vi "EditOptions.vi"(8 "error in":errorcluster, 11 "node in":refnum<class "CEF_serializable node folder.lvclass">=refnum) -> (0 "error out":errorcluster, 1 "edit options":T1, 2 "subnodes class":T2, 3 "node out":refnum<class "CEF_serializable node folder.lvclass">)   [LabVIEW 2025, in "CEF_serializable node folder.lvclass"]
doc: "Contains the options for the Menu that will be displayed when doing right click on an item.\nThe sub nodes class configures which nodes can be added to this nodes\nAnd the edit options determine which options are available for the node.\nThis configuration is stored in this VI in case some dynamic configuration is required for the menu options or sub nodes.\nCopyright 2017 National Instruments Corporation\n\nLicensed under the Apache License, Version 2.0 (the \"License\"); you may not use this file except in compliance with the License. You may obtain a copy of the License at http://www.apache.org/licenses/LICENSE-2.0\nUnless required by applicable law or agreed to in writing, software distributed under the License is distributed on an \"AS IS\" BASIS, WITHOUT WARRANTIES OR CONDITIONS OF ANY KIND, either express or implied. See the License for the specific language governing permissions and limitations under the License."
uses:
  CEF_serializable node folder.lvclass
  CEF_serializable node folder.lvclass/CEF_serializable node folder.ctl
  <vilib>/NI/Configuration Framework/Node/NISE_CEF_Node.lvclass
  <vilib>/NI/Configuration Framework/Node/NodeMenuOptions.ctl
  <vilib>/NI/Configuration Framework/Node/SubNodeCluster.ctl
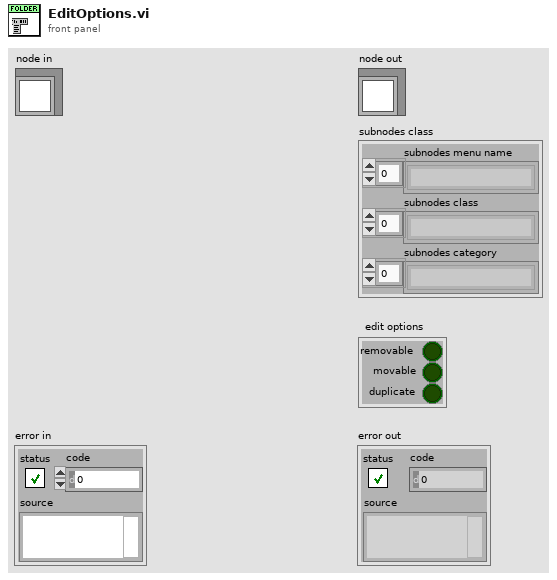
[diagram p1: front panel]
types:
  T1 = typedef "NISE_CEF_Node.lvclass/NodeMenuOptions.ctl" = cluster{"removable":bool, "movable":bool, "duplicate":bool}
  T2 = typedef "NISE_CEF_Node.lvclass/SubNodeCluster.ctl" = cluster{"subnodes menu name":string[], "subnodes class":string[], "subnodes category":string[]}
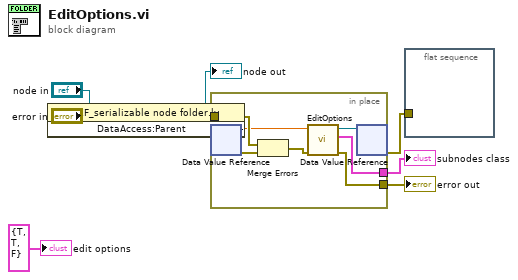
[diagram p0: block diagram]
diagram:
  n1 = property class="CEF_serializable node folder.lv"(reference="node in", error in="error in") -> (reference out=→"node out":refnum<class "CEF_serializable node folder.lvclass">, error out=w9:errorcluster, "DataAccess:Parent"=w8)
  n2 = in-place {
    in-place-border: w9 -> [w16]
    in-place-border: [w15] -> w4
    in-place-border: [w10] -> w2
    n3 = in-place-dvr #1(w8) -> (w14:dbl, w11:errorcluster)
    n4 = Merge Errors(w16, w11) -> (w12:errorcluster)
    n5 = call-dynamic "EditOptions.vi"("error in"=w12, "node in"=w14) -> ("error out"=w15:errorcluster, "subnodes class"=w10:T2, "node out"=w13:refnum<class "NISE_CEF_Node.lvclass">)  [unwired: 6 in, 1 out]
    n6 = in-place-dvr #1(w13) -> (w7:errorcluster)  [unwired: 1 out]
  }
  "error out" <- w4
  "subnodes class" <- w2
  n7 = flat-sequence {
    tunnel: w7 -> [_]
    frame #0 {
    }
  }
  "edit options" <- T1 {"removable"=TRUE, "movable"=TRUE, "duplicate"=FALSE} ("edit options")
